vi "RSZVB Set Sweep Segment Start Frequency.vi"(7 "Start Frequency (0.0 Hz)":dbl format="%^.3e", 8 "error in (no error)":errorcluster {"code" format="%.0x"}, 9 "Segment (1)":i32=1, 10 "Channel (1)":i32=1, 11 "VISA session":refnum<visa-resource-name>) -> (0 "error out":errorcluster {"code" format="%.0x"}, 3 "dup VISA session":refnum<visa-resource-name>)   [LabVIEW 2011]
doc: "This VI defines the Start frequency of sweep segment no. <Segment>.\n\nRemote-control command(s):\n[SENSe<Ch>:]SEGMent<Seg>:FREQuency:STARt"
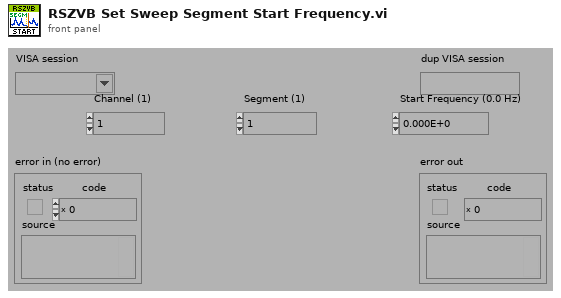
[diagram p1: front panel]
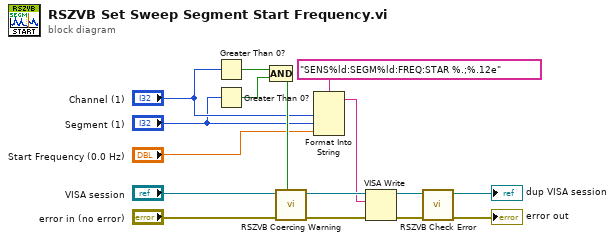
[diagram p0: block diagram]
diagram:
  n1 = Greater Than 0?(x="Channel (1)") -> (x > 0?=w9:bool)
  n2 = Greater Than 0?(x="Segment (1)") -> (x > 0?=w8:bool)
  n3 = Compound Arithmetic op=AND(w9, w8) -> (w11:bool)
  n4 = call "RSZVB Coercing Warning.vi"("In Range?"=w11, "error in (no error)"="error in (no error)", "VISA session"="VISA session") -> ("error out"=w14:errorcluster, "dup VISA session"=w15:refnum<visa-resource-name>)  [unwired: 7 in]
  n5 = Format Into String(format string="SENS%ld:SEGM%ld:FREQ:STAR %.;%.12e", "Channel (1)", "Segment (1)", "Start Frequency (0.0 Hz)") -> (resulting string=w10:string)  [unwired: 2 in, 1 out]
  n6 = VISA Write(VISA resource name=w15, write buffer=w10, error in (no error)=w14) -> (VISA resource name out=w12:refnum<visa-resource-name>, error out=w13:errorcluster)  [unwired: 1 out]
  n7 = call "RSZVB Check Error.vi"("error in (no error)"=w13, "VISA session"=w12) -> ("error out"=→"error out":errorcluster, "dup VISA session"=→"dup VISA session":refnum<visa-resource-name>)  [unwired: 8 in]
